vi "XY Graph Load Plot(s) from ASCII File.vi"(7 "Header Definitions":T2, 8 "error in (no error)":errorcluster, 10 "Delimiter (TAB)":string="\t", 11 "File Path":path) -> (0 "error out":errorcluster, 1 "Plot Scales Array":T1[](array[typedef]), 2 "Plot Name Array":string[](array[string]), 3 "Plot Array":cluster{"X Array":dbl[], "Y Array":dbl[]}[](array[cluster]))   [LabVIEW 2019, in "XY Graph Add-Ons.lvlib"]
uses:
  XY Graph Add-Ons.lvlib
  ASCII File Header Definition.ctl
  Plot Scale Labels.ctl
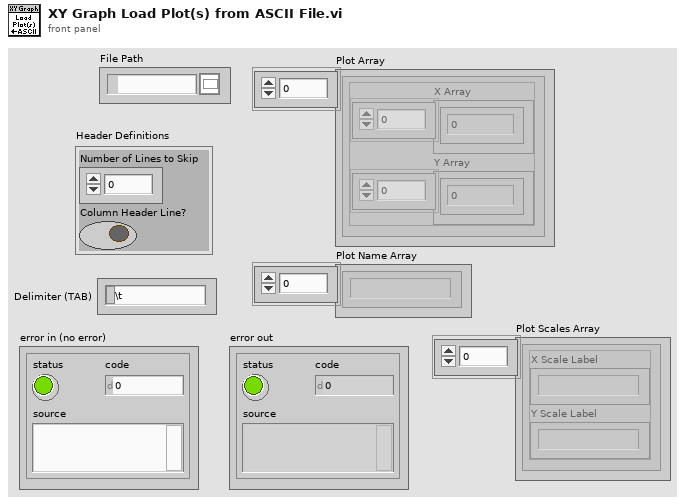
[diagram p1: front panel]
types:
  T1 = typedef "Plot Scale Labels.ctl" = cluster{"X Scale Label":string, "Y Scale Label":string}
  T2 = typedef "ASCII File Header Definition.ctl" = cluster{"Number of Lines to Skip":i32, "Column Header Line?":bool}
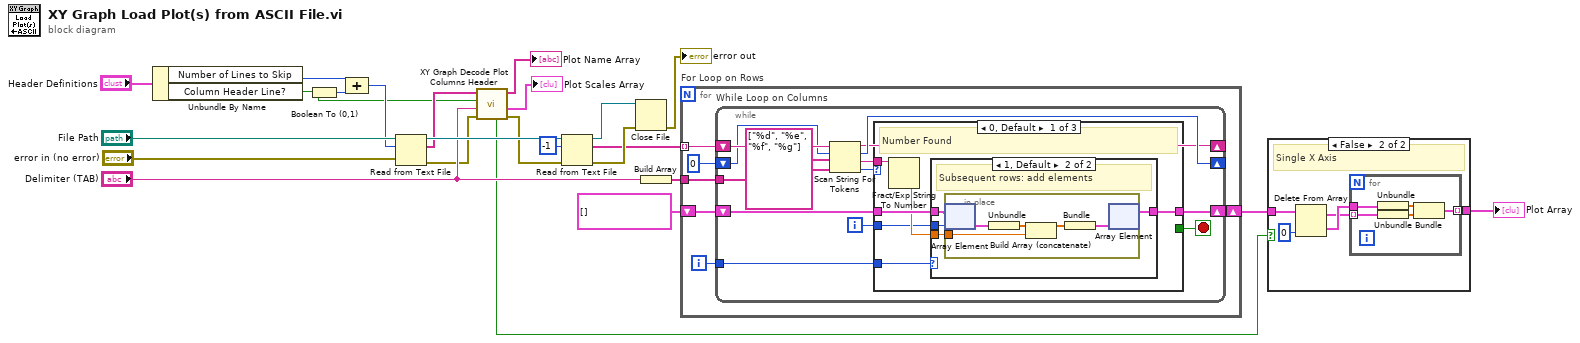
[diagram p0: block diagram]
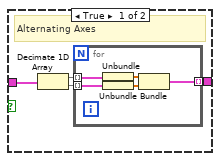
[diagram p2: hidden frame]
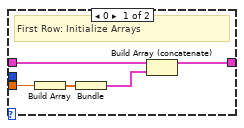
[diagram p3: hidden frame]
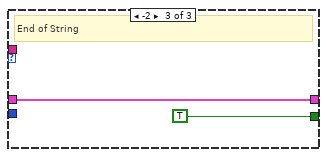
[diagram p5: hidden frame]
diagram:
  n1 = Unbundle By Name("Header Definitions") -> ("Number of Lines to Skip"=w22:i32, "Column Header Line?"=w5:bool)
  n2 = Boolean To (0,1)(Boolean=w5) -> (0, 1=w21:i16)
  n3 = Compound Arithmetic op=ADD(w22, w21) -> (w20:i32)
  n4 = Read from Text File(file (use dialog)="File Path", count=w20, error in="error in (no error)") -> (refnum out=w18:refnum<file>, text=w12:string[], error out=w7:errorcluster)  [unwired: 1 in, 1 out]
  n5 = call "XY Graph Decode Plot Columns Header.vi"("Error In"=w7, "Delimiter"="Delimiter (TAB)", "Column Header Line? (F)"=w5, "Header String Array"=w12) -> ("Error Out"=w6:errorcluster, "Plot Scales Array"=→"Plot Scales Array":T1[], "Plot Name Array"=→"Plot Name Array":string[], "Alternating Axes?"=w1:bool)  [unwired: 4 in]
  n6 = Read from Text File(file (use dialog)=w18, count=-1, error in=w6) -> (refnum out=w15:refnum<file>, text=w14:string[], error out=w16:errorcluster)  [unwired: 1 in, 1 out]
  n7 = Close File(refnum=w15, error in=w16) -> (error out=→"error out":errorcluster)  [unwired: 1 out]
  n8 = Build Array("Delimiter (TAB)") -> (w13:string[])
  n9 = for "For Loop on Rows" {
    tunnel: w14 -> [w30] mode=indexing
    tunnel: w13 -> [w29]
    shift-right: [w26] -> w10
    shift-left: cluster{dbl[]}[] [] -> [w27]
    i -> [w25]
    n10 = while "While Loop on Columns" {
      tunnel: w29 -> [w42]
      shift-right: [w38] -> _
      shift-left: w30 -> [w43]
      shift-right: [w39] -> _
      shift-left: 0 ("offset past token") -> [w40]
      shift-right: [w32] -> w26
      shift-left: w27 -> [w34]
      tunnel: w25 -> [w31]
      i -> [w33]
      stop <- w35 stop-if-true
      n11 = Scan String For Tokens(6:w42, 7:string[] ["%d", "%e", "%f", "%g"] ("operators (none)"), 8:w40, 9:w43) -> (0:w37:i32, 1:w36:string, 2:w39:i32, 3:w38:string)  [unwired: 2 in]
      n12 = case shown="0, Default" w37 {
        tunnel: w36 -> [w49 _ _]
        tunnel: [_ _ TRUE] -> w35
        tunnel: w34 -> [w48 w64 w65]
        tunnel: w33 -> [w45 _ _]
        tunnel: [w46 w64 w65] -> w32
        tunnel: w31 -> [w44 _ _]
        frame 0, Default {
          # "Number Found"
          n13 = Fract/Exp String To Number(string=w49) -> (number=w47:dbl)  [unwired: 3 in, 1 out]
          n14 = case shown="1, Default" w44 {
            tunnel: w48 -> [w52 w58]
            tunnel: w47 -> [w54 w57]
            tunnel: [w50 w56] -> w46
            tunnel: w45 -> [_ w55]
            frame 0 {
              # "First Row: Initialize Arrays"
              n15 = Build Array(w54) -> (w53:dbl[])
              n16 = Bundle(w53) -> (w51:cluster{dbl[]})  [unwired: 1 in]
              n17 = Build Array (concatenate)(w52, w51) -> (w50:cluster{dbl[]}[])
            }
            frame 1, Default {
              # "Subsequent rows: add elements"
              n18 = in-place {
                in-place-border: w57 -> [w62]
                n19 = in-place-array #1(w58, w55) -> (w63:cluster{dbl[]})
                n20 = Unbundle(w63) -> (w60:dbl[])
                n21 = Build Array (concatenate)(w60, w62) -> (w61:dbl[])
                n22 = Bundle(w61) -> (w59:cluster{dbl[]})  [unwired: 1 in]
                n23 = in-place-array #1(w59) -> (w56:cluster{dbl[]}[])  [unwired: 1 out]
              }
            }
          }
        }
        frame -1 {
          # "Some columns have less numbers than others"
          # "Number not Found"
        }
        frame -2 {
          # "End of String"
        }
      }
    }
  }
  n24 = case shown="False" w1 {
    tunnel: w10 -> [w70 w79]
    tunnel: [w67 w80] -> w9
    frame True {
      # "Alternating Axes"
      n25 = Decimate 1D Array(w70) -> (w69:cluster{dbl[]}[], w68:cluster{dbl[]}[])
      n26 = for {
        tunnel: w69 -> [w75] mode=indexing
        tunnel: w68 -> [w74] mode=indexing
        tunnel: [w71] -> w67 mode=indexing
        n27 = Unbundle(w75) -> (w73:dbl[])
        n28 = Unbundle(w74) -> (w72:dbl[])
        n29 = Bundle(w73, w72) -> (w71:cluster{dbl[], dbl[]})  [unwired: 1 in]
      }
    }
    frame False {
      # "Single X Axis"
      n30 = Delete From Array(array=w79, index=0) -> (deleted portion=w77:cluster{dbl[]}, array with subset deleted=w76:cluster{dbl[]}[])  [unwired: 1 in]
      n31 = for {
        tunnel: w77 -> [w85]
        tunnel: w76 -> [w84] mode=indexing
        tunnel: [w81] -> w80 mode=indexing
        n32 = Unbundle(w85) -> (w83:dbl[])
        n33 = Unbundle(w84) -> (w82:dbl[])
        n34 = Bundle(w83, w82) -> (w81:cluster{dbl[], dbl[]})  [unwired: 1 in]
      }
    }
  }
  "Plot Array" <- w9
